vi "InterpolateCalibration.vi"(1 "Input":dbl, 2 "Calibration Data":dbl[][](array[numeric])) -> (0 "Interpolated Output":dbl)   [LabVIEW 2019]
uses:
  <vilib>/gmath/NI_Gmath.lvlib
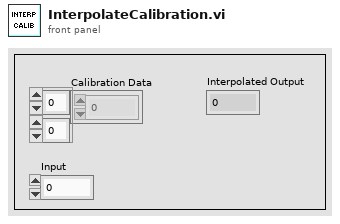
[diagram p1: front panel]
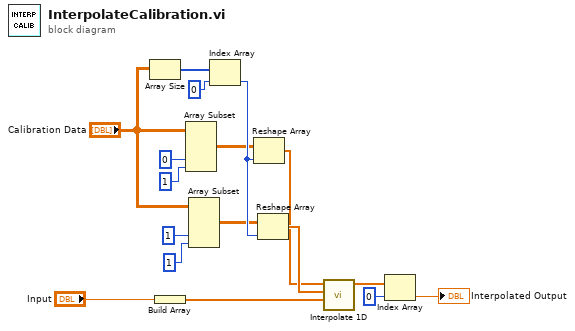
[diagram p0: block diagram]
diagram:
  n1 = Array Size(array="Calibration Data") -> (size(s)=w13:i32[])
  n2 = Build Array("Input") -> (w3:dbl[])
  n3 = Array Subset(array="Calibration Data", index (col)=0 ("index"), length (col)=1 ("length")) -> (w9:dbl[][])  [unwired: 2 in]
  n4 = Array Subset(array="Calibration Data", index (col)=1 ("index"), length (col)=1 ("length")) -> (w14:dbl[][])  [unwired: 2 in]
  n5 = Index Array(array=w13, index=0) -> (element=w16:i32)
  n6 = Reshape Array(w9, w16) -> (w10:dbl[])
  n7 = Reshape Array(w14, w16) -> (w15:dbl[])
  n8 = call <vilib>:"Interpolate 1D.vi"("xi"=w3, "X"=w15, "Y"=w10) -> ("yi"=w2:dbl[])  [unwired: 6 in, 2 out]
  n9 = Index Array(array=w2, index=0) -> (element=→"Interpolated Output":dbl)
